vi "Wavelength to Grating Position.vi"(5 "grating index (0)":u8, 7 "turret index (0)":u8, 8 "error in (no error)":errorcluster, 10 "wavelength, nm":dbl, 11 "SOL MS in":refnum<class "PL SOL Instruments MS.lvclass">) -> (0 "error out":errorcluster, 2 "grating position":i32, 3 "SOL MS out":refnum<class "PL SOL Instruments MS.lvclass">)   [LabVIEW 2015, in "PL SOL Instruments MS.lvclass"]
doc: "Converts <b>wavelength</b> of the specified <b>grating</b> of the specified <b>turret</b> to <b>grating position</b>."
uses:
  PL SOL Instruments MS.lvclass
  PL SOL Instruments MS.lvclass/PL SOL Instruments MS.ctl
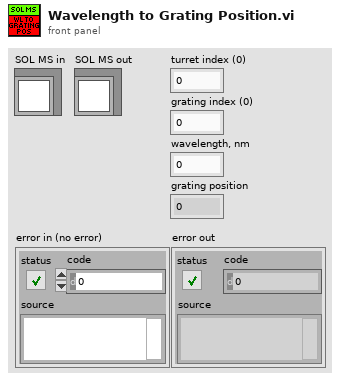
[diagram p1: front panel]
types:
  T1 = cluster{"name":string, "step timeout, ms":u32, "reset timeout, ms":u32, "gratings":cluster{"name":string, "step timeout, ms":u32, "reset timeout, ms":u32, "turret position":i32, "reset position":i32, "max position":i32, "backlash distance":i32, "step size, rad":dbl, "groove density, g/mm":dbl, "theta2, rad":dbl, "blaze wavelength, nm":dbl, "focal length, cm":dbl, "manual change":bool, "manual change position":i32}[], "current grating":cluster{"index":u8, "position":i32}}[]
  T2 = cluster{"name":string, "step timeout, ms":u32, "reset timeout, ms":u32, "gratings":cluster{"name":string, "step timeout, ms":u32, "reset timeout, ms":u32, "turret position":i32, "reset position":i32, "max position":i32, "backlash distance":i32, "step size, rad":dbl, "groove density, g/mm":dbl, "theta2, rad":dbl, "blaze wavelength, nm":dbl, "focal length, cm":dbl, "manual change":bool, "manual change position":i32}[], "current grating":cluster{"index":u8, "position":i32}}
  T3 = cluster{"name":string, "step timeout, ms":u32, "reset timeout, ms":u32, "turret position":i32, "reset position":i32, "max position":i32, "backlash distance":i32, "step size, rad":dbl, "groove density, g/mm":dbl, "theta2, rad":dbl, "blaze wavelength, nm":dbl, "focal length, cm":dbl, "manual change":bool, "manual change position":i32}[]
  T4 = cluster{"name":string, "step timeout, ms":u32, "reset timeout, ms":u32, "turret position":i32, "reset position":i32, "max position":i32, "backlash distance":i32, "step size, rad":dbl, "groove density, g/mm":dbl, "theta2, rad":dbl, "blaze wavelength, nm":dbl, "focal length, cm":dbl, "manual change":bool, "manual change position":i32}
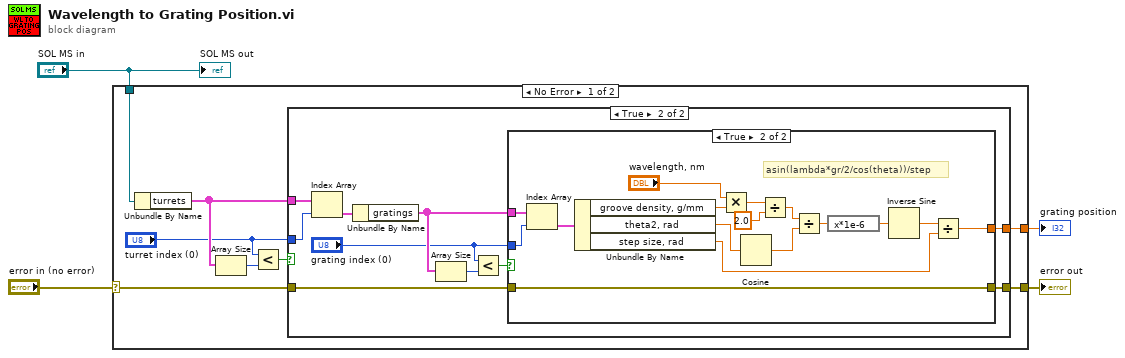
[diagram p0: block diagram]
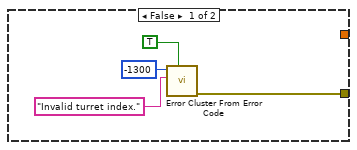
[diagram p2: hidden frame]
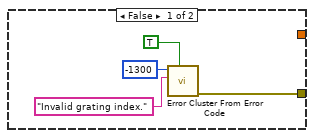
[diagram p3: hidden frame]
diagram:
  n1 = case shown="No Error" "error in (no error)" {
    selector: "error in (no error)" -> [w6 w47]
    tunnel: "SOL MS in" -> [w12 _]
    tunnel: [w11 _] -> w1
    tunnel: [w7 w47] -> w2
    frame No Error {
      n2 = Unbundle By Name(w12) -> ("turrets"=w10:T1)
      n3 = Array Size(array=w10) -> (size(s)=w9:i32)
      n4 = Less?(x="turret index (0)", y=w9) -> (x < y?=w8:bool)
      n5 = case shown="True" w8 {
        tunnel: w10 -> [_ w26]
        tunnel: [_ w24] -> w11
        tunnel: [w13 w20] -> w7
        tunnel: w6 -> [_ w18]
        tunnel: "turret index (0)" -> [_ w19]
        frame False {
          n6 = call <vilib>:"Error Cluster From Error Code.vi"("show call chain? (False)"=TRUE, "error message (\"\")"="Invalid turret index." ("error message (\"\")"), "error code (0)"=-1300) -> ("error out"=w13:errorcluster)  [unwired: 6 in]
        }
        frame True {
          n7 = Index Array(array=w26, index=w19) -> (element=w25:T2)
          n8 = Unbundle By Name(w25) -> ("gratings"=w22:T3)
          n9 = Array Size(array=w22) -> (size(s)=w23:i32)
          n10 = Less?(x="grating index (0)", y=w23) -> (x < y?=w21:bool)
          n11 = case shown="True" w21 {
            tunnel: w22 -> [_ w46]
            tunnel: "grating index (0)" -> [_ w45]
            tunnel: [_ w31] -> w24
            tunnel: [w27 w44] -> w20
            tunnel: w18 -> [_ w44]
            frame False {
              n12 = call <vilib>:"Error Cluster From Error Code.vi"("show call chain? (False)"=TRUE, "error message (\"\")"="Invalid grating index." ("error message (\"\")"), "error code (0)"=-1300) -> ("error out"=w27:errorcluster)  [unwired: 6 in]
            }
            frame True {
              # "asin(lambda*gr/2/cos(theta))/step"
              n13 = Index Array(array=w46, index=w45) -> (element=w32:T4)
              n14 = Unbundle By Name(w32) -> ("groove density, g/mm"=w33:dbl, "theta2, rad"=w37:dbl, "step size, rad"=w42:dbl)
              n15 = Multiply(x="wavelength, nm", y=w33) -> (x*y=w34:dbl)
              n16 = Cosine(x=w37) -> (cos(x)=w38:dbl)
              n17 = Divide(x=w34, y=2.0) -> (x/y=w36:dbl)
              n18 = Divide(x=w36, y=w38) -> (x/y=w39:dbl)
              n19 = expression code="x*1e-6"(w39) -> (w40:dbl)
              n20 = Inverse Sine(1:w40) -> (0:w41:dbl)
              n21 = Divide(x=w41, y=w42) -> (x/y=w31:dbl)
            }
          }
        }
      }
    }
    frame Error {
    }
  }
  "grating position" <- w1
  "error out" <- w2
  "SOL MS out" <- "SOL MS in"
